vi "getEnabled.vi"(0 "Interface in":T1, 11 "error in (no error)":errorcluster) -> (4 "Interface out":T1, 6 "Enabled":u8 format="%.0x", 15 "error out":errorcluster)   [LabVIEW 2017, in "BuckBoostInterface.lvlib"]
uses:
  BuckBoostInterface.lvlib
  Interface.ctl
  <instrlib>/_niInstr/Instruction Framework/v1/Host/Instruction Target/niInstr Instruction Target v1 Host.lvclass
  <instrlib>/_niInstr/Instruction Framework/v1/Host/Instruction Framework Context/niInstr Instruction Framework Context v1 Host.lvclass
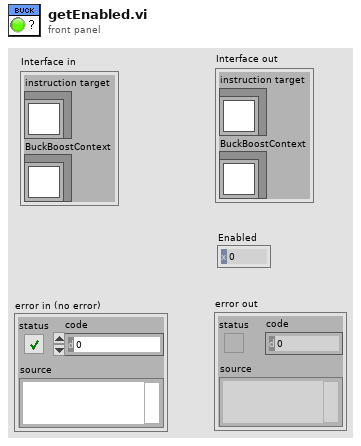
[diagram p1: front panel]
types:
  T1 = typedef "BuckBoostInterface.lvlib/Interface.ctl" = cluster{"instruction target":refnum<class "niInstr Instruction Target v1 Host.lvclass">, "BuckBoostContext":refnum<class "niInstr Instruction Framework Context v1 Host.lvclass">}
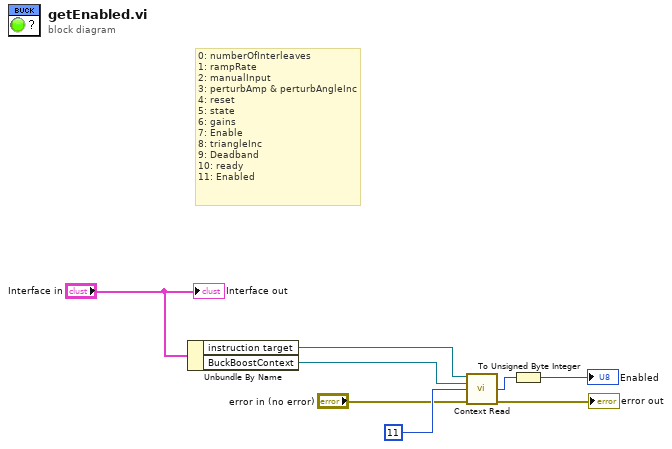
[diagram p0: block diagram]
diagram:
  # "0: numberOfInterleaves\n1: rampRate\n2: manualInput\n3: perturbAmp & perturbAngleInc\n4: reset\n5: state\n6: gains\n7: Enable\n8: triangleInc\n9: Deadband\n10: ready\n11: Enabled"
  n1 = Unbundle By Name("Interface in") -> ("instruction target"=w5:refnum<class "niInstr Instruction Target v1 Host.lvclass">, "BuckBoostContext"=w4:refnum<class "niInstr Instruction Framework Context v1 Host.lvclass">)
  n2 = call <instrlib>:"Context Read.vi"("instruction target in"=w5, "context in"=w4, "address"=u64 11, "error in"="error in (no error)") -> ("data"=w2:u64, "error out"=→"error out":errorcluster)  [unwired: 8 in, 2 out]
  n3 = To Unsigned Byte Integer(number=w2) -> (unsigned 8bit integer=→"Enabled":u8)
  "Interface out" <- "Interface in"
